vi "Create UDP.vi"(8 "error in (no error)":errorcluster, 9 "PCL Decimation":u16, 10 "Protocol Properties":T1, 11 "Target in":refnum<k24>) -> (0 "error out":errorcluster, 2 "Instrument Addon Custom Device refnum":T2=18446744073709551615 format="%.0x", 3 "Target out":refnum<k24>)   [LabVIEW 2019, in "Scripting API.lvlib"]
uses:
  Scripting API.lvlib
  NationalInstruments.VeriStand.SystemDefinitionAPI
  <vilib>/NI VeriStand/Custom Device API/Custom Device Item Ref.ctl
  <vilib>/NI VeriStand/Custom Device API/Custom Device API.lvlib
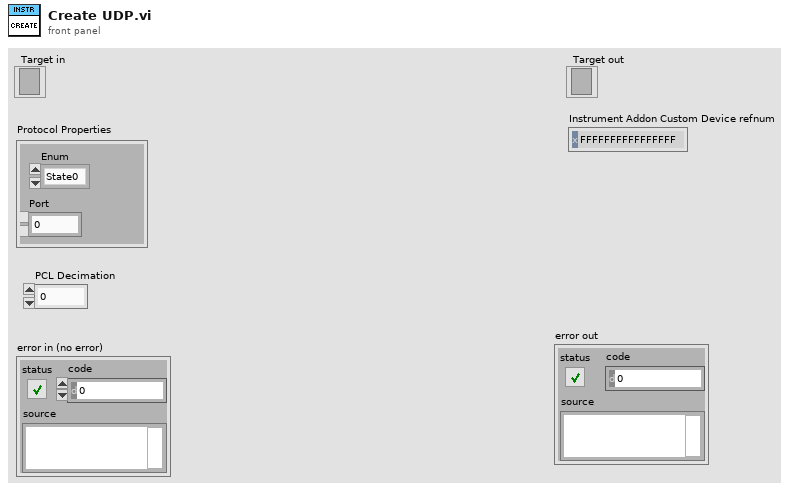
[diagram p1: front panel]
types:
  T1 = cluster{"Port":dbl, "Enum":enum16{"State0", "State1"}}
  T2 = typedef "Custom Device API.lvlib/Custom Device Item Ref.ctl" = u64
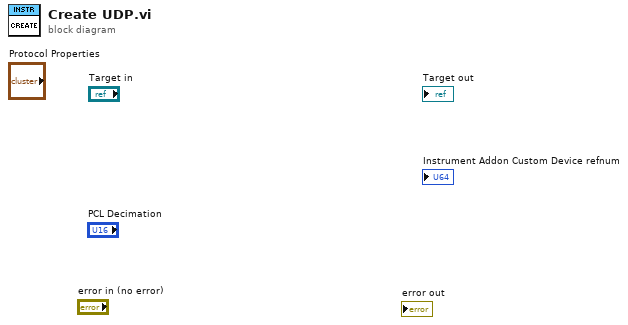
[diagram p0: block diagram]
diagram:
